vi "openXMLFile.vi"(8 "error in (no error)":errorcluster, 10 "Path":path) -> (0 "error out":errorcluster, 3 "NativeXML out":refnum<class "NativeXML.lvclass">)   [LabVIEW 2011, in "Tools.lvlib" / "xml.lvlib" / "NativeXML.lvclass"]
uses:
  NativeXML.lvclass
  NativeXML.lvclass/NativeXML.ctl
  <vilib>/xml/Load XML File.vi
  <vilib>/xml/NI_XML.lvlib
  Program Files/National Instruments/LabVIEW 2011/resource/objmgr/DOMUserDefRef.rc
panel:
  out "xmlString":string
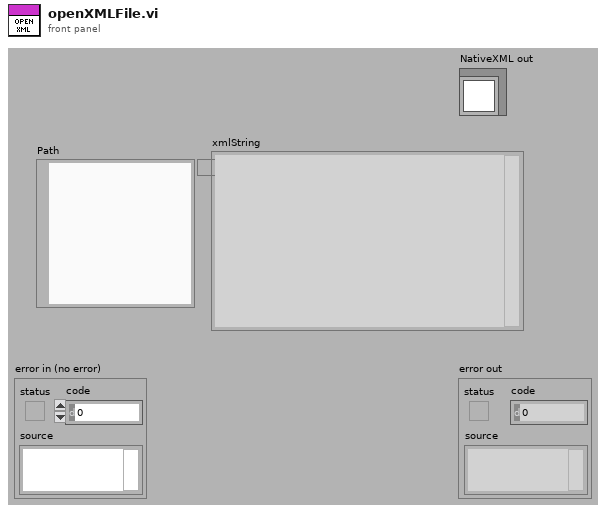
[diagram p1: front panel]
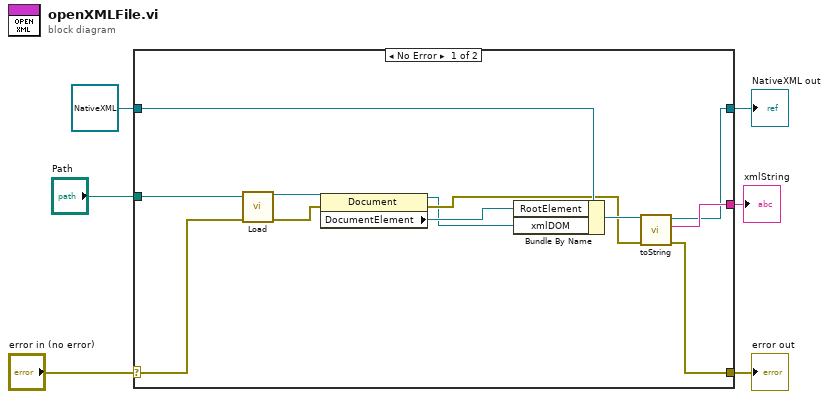
[diagram p0: block diagram]
diagram:
  n1 = case shown="No Error" "error in (no error)" {
    selector: "error in (no error)" -> [w18 w20]
    tunnel: [w11 w20] -> w5
    tunnel: [w12 w19] -> w3
    tunnel: refnum<class "NativeXML.lvclass"> refnum ("NativeXML in") -> [w16 w19]
    tunnel: "Path" -> [w17 _]
    tunnel: [w13 _] -> w1
    frame No Error {
      n2 = call-poly <vilib>:"Load.vi"("path to XML document"=w17, "error in (no error)"=w18) -> ("DOM document out"=w10:refnum<k20>, "error out"=w9:errorcluster)  [unwired: 11 in, 1 out]
      n3 = property class="Document"(reference=w10, error in=w9) -> (reference out=w7:refnum<k20>, error out=w8:errorcluster, "DocumentElement"=w15:refnum<k20>)
      n4 = Bundle By Name(cluster=w16, "RootElement"=w15, "xmlDOM"=w7) -> (w14:refnum<class "NativeXML.lvclass">)
      n5 = call "toString.vi"("error in (no error)"=w8, "NativeXML in"=w14) -> ("error out"=w11:errorcluster, "xmlString"=w13:string, "NativeXML out"=w12:refnum<class "NativeXML.lvclass">)  [unwired: 7 in]
    }
    frame Error {
    }
  }
  "error out" <- w5
  "NativeXML out" <- w3
  "xmlString" <- w1
